vi "List Roots Priv.vi"(8 "error in":errorcluster, 11 "Tree Dict":variant) -> (0 "error out":errorcluster, 1 "Root Names":string[](array[string]), 2 "Root IDs":string[](array[string]), 3 "Tree Dict":variant)   [LabVIEW 2020, in "NI_VIAnCFGDataStructure.lvlib" / "Tree.lvclass"]
uses:
  <vilib>/addons/analyzer/VIAnCFGDataStructure/Tree Manager/Tree.lvclass
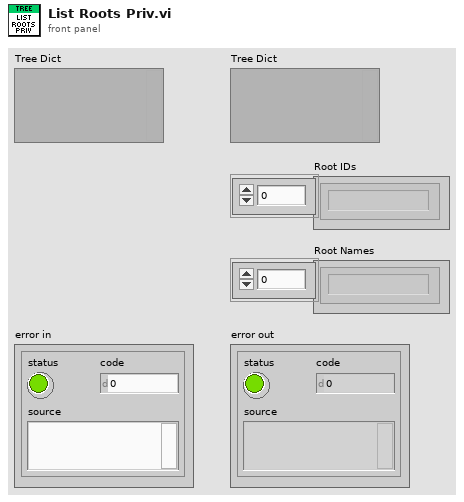
[diagram p1: front panel]
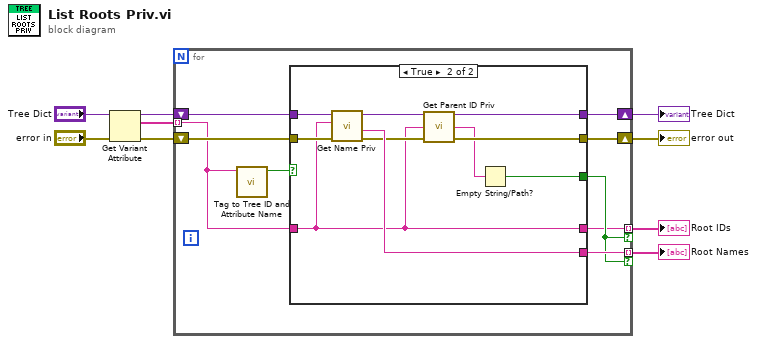
[diagram p0: block diagram]
diagram:
  n1 = Get Variant Attribute(Variant="Tree Dict", error in="error in") -> (duplicate Variant=w3:variant, names=w7:string[], error out=w5:errorcluster)  [unwired: 2 in, 1 out]
  n2 = for {
    shift-right: [w18] -> w4
    shift-left: w3 -> [w16]
    shift-right: [w17] -> w6
    shift-left: w5 -> [w15]
    tunnel: w7 -> [w12] mode=indexing
    tunnel: [w10] -> w8 mode=indexing if=w13
    tunnel: [w14] -> w9 mode=indexing if=w13
    n3 = call <vilib>:"Tag to Tree ID and Attribute Name.vi"("Tag"=w12) -> ("Tree"=w11:bool)  [unwired: 8 in, 2 out]
    n4 = case shown="True" w11 {
      tunnel: [w20 w30] -> w18
      tunnel: [w19 w29] -> w17
      tunnel: w16 -> [w20 w27]
      tunnel: w15 -> [w19 w26]
      tunnel: [_ w25] -> w14
      tunnel: [_ w24] -> w13
      tunnel: w12 -> [_ w21]
      tunnel: [_ w21] -> w10
      frame False {
      }
      frame True {
        n5 = call <vilib>:"Get Name Priv.vi"("error in"=w26, "Unique ID"=w21, "Tree Dictionary"=w27) -> ("error out"=w22:errorcluster, "Name"=w25:string, "Tree Dictionary Out"=w23:variant)  [unwired: 6 in]
        n6 = call <vilib>:"Get Parent ID Priv.vi"("Tree Dictionary"=w23, "Unique ID"=w21, "error in"=w22) -> ("Tree Dictionary Out"=w30:variant, "Parent ID"=w28:string, "error out"=w29:errorcluster)  [unwired: 10 in]
        n7 = Empty String/Path?(string/path=w28) -> (empty?=w24:bool)
      }
    }
  }
  "Root Names" <- w9
  "Root IDs" <- w8
  "error out" <- w6
  "Tree Dict" <- w4
